vi "high score pattern.vi"(4 "error in \n(diody gora)":errorcluster, 5 "task in\n(diody dol)":refnum<k21>, 6 "error in\n(diody dol)":errorcluster, 7 "task in \n(diody gora)":refnum<k21>) -> (0 "error out\n(diody dolne)":errorcluster, 1 "task out\n(diody dolne)":refnum<k21>, 2 "error out\n(diody gorne)":errorcluster, 3 "task out\n(diody gorne)":refnum<k21>)   [LabVIEW 2023]
uses:
  <vilib>/DAQmx/write.llb/DAQmx Write (Digital 1D Bool 1Chan 1Samp).vi
  <vilib>/DAQmx/miscellaneous.llb/DAQmx Fill In Error Info.vi
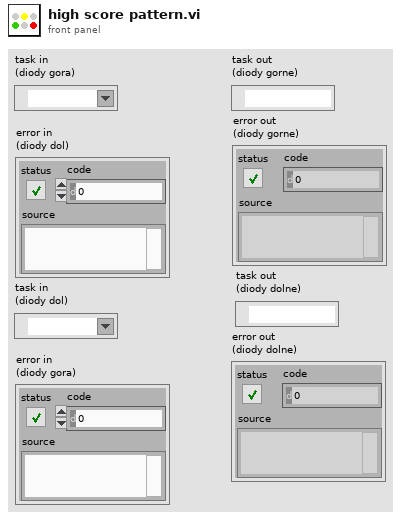
[diagram p1: front panel]
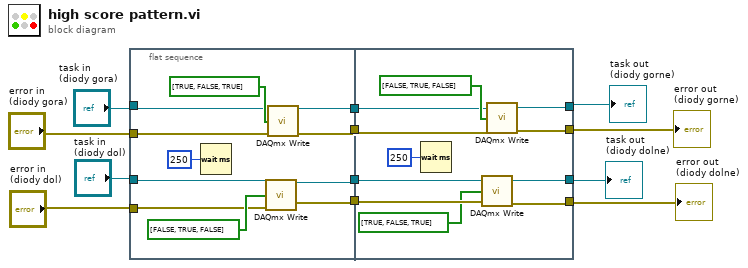
[diagram p0: block diagram]
diagram:
  n1 = flat-sequence {
    tunnel: [w23] -> w12
    tunnel: [w22] -> w11
    tunnel: "task in\n(diody dol)" -> [w18]
    tunnel: "task in \n(diody gora)" -> [w17]
    tunnel: [w16] -> w10
    tunnel: [w15] -> w9
    tunnel: "error in\n(diody dol)" -> [w14]
    tunnel: "error in \n(diody gora)" -> [w13]
    tunnel: w12 -> [w33]
    tunnel: w11 -> [w34]
    tunnel: [w31] -> w6
    tunnel: [w27] -> w5
    tunnel: [w30] -> w4
    tunnel: w10 -> [w26]
    tunnel: w9 -> [w25]
    tunnel: [w24] -> w7
    frame #0 {
      n2 = Wait (ms)(milliseconds to wait=u32 250) -> ()  [unwired: 1 out]
      n3 = call-poly <vilib>:"DAQmx Write.vi"("task/channels in"=w18, "data"=bool[] [FALSE, TRUE, FALSE], "error in"=w14) -> ("task out"=w22:refnum<k21>, "error out"=w23:errorcluster)  [unwired: 10 in, 1 out]
      n4 = call-poly <vilib>:"DAQmx Write.vi"("task/channels in"=w17, "data"=bool[] [TRUE, FALSE, TRUE], "error in"=w13) -> ("task out"=w16:refnum<k21>, "error out"=w15:errorcluster)  [unwired: 10 in, 1 out]
    }
    frame #1 {
      n5 = Wait (ms)(milliseconds to wait=u32 250) -> ()  [unwired: 1 out]
      n6 = call-poly <vilib>:"DAQmx Write.vi"("task/channels in"=w34, "data"=bool[] [TRUE, FALSE, TRUE], "error in"=w33) -> ("task out"=w31:refnum<k21>, "error out"=w27:errorcluster)  [unwired: 10 in, 1 out]
      n7 = call-poly <vilib>:"DAQmx Write.vi"("task/channels in"=w26, "data"=bool[] [FALSE, TRUE, FALSE], "error in"=w25) -> ("task out"=w30:refnum<k21>, "error out"=w24:errorcluster)  [unwired: 10 in, 1 out]
    }
  }
  "error out\n(diody gorne)" <- w7
  "task out\n(diody dolne)" <- w6
  "error out\n(diody dolne)" <- w5
  "task out\n(diody gorne)" <- w4
